vi "t0_Valid.vi"(3 "T0":timestamp) -> (1 "Valid":bool)   [LabVIEW 2025]
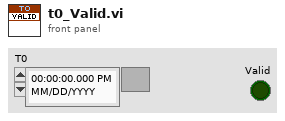
[diagram p1: front panel]
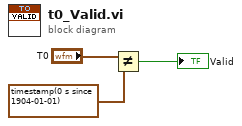
[diagram p0: block diagram]
diagram:
  n1 = Not Equal?(x="T0", y=timestamp(0 s since 1904-01-01)) -> (x != y?=→"Valid":bool)
